vi "Dashboard custom_bartender&global&gripper&camera.vi"() -> ()   [LabVIEW 2017]
uses:
  C:/Users/IMR Lab/Documents/LabVIEW Data/UniversalRobotsSDK_LABView/LabVIEW/Examples/LabVIEW10/UnderAutomation.UniversalRobots.dll
  UnderAutomation.UniversalRobots.dll
  Global 1.vi
panel:
  out "RZ_havetogo":string
  out "RY_havetogo":string
  out "RX_havetogo":string
  out "Z_havetogo":string
  out "Y_havetogo":string
  out "X_havetogo":string
  out "data out":string
  out "TCPOffsetRZ":dbl
  out "TCPOffsetRY":dbl
  out "TCPOffsetRX":dbl
  out "TCPOffsetZ":dbl
  out "TCPOffsetY":dbl
  out "TCPOffsetX":dbl
  out "3rd Order":bool
  out "2nd Order":bool
  out "1st Order":bool
  in  "stop":bool
  in  "TCP switch (server)":bool
  out "Rx":dbl
  out "Rz":dbl
  out "Ry":dbl
  out "Enabled":bool
  out "Port":i32
  in  "Move to particular posture":bool
  in  "Move to Zero position":bool
  out "Connected":bool
  in  "Robot IP(192.168.112.182)":string
  out "Connect error":errorcluster
  in  "Power on\nRelease brake":bool
  in  "Power off":bool
  in  "Connect":bool
  in  "Send script":bool
  in  "Script to execute":string
  out "Powered on":bool
  out "X":dbl
  out "Y":dbl
  out "Z":dbl
  out "License state":string
  # "movel(p[-0.0753945, -0.304532, 0.314608, -0.194623, 2.71667, -1.00228], a= 0.5, v=0.25)"
  # "movej( get_inverse_kin(p[0.3138, 0.0814, 0.1647, 0.4226, -2.3876, -2.3851]),  a=0.5, v=0.25, t=0, r=0)"
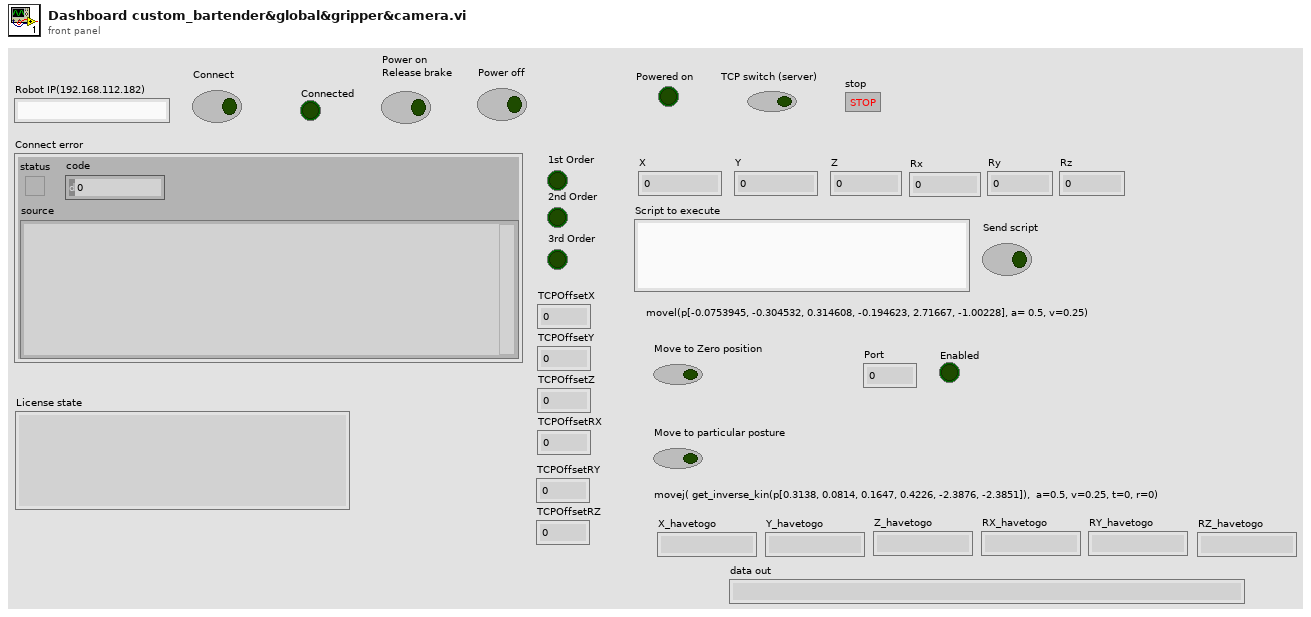
[diagram p1: front panel]
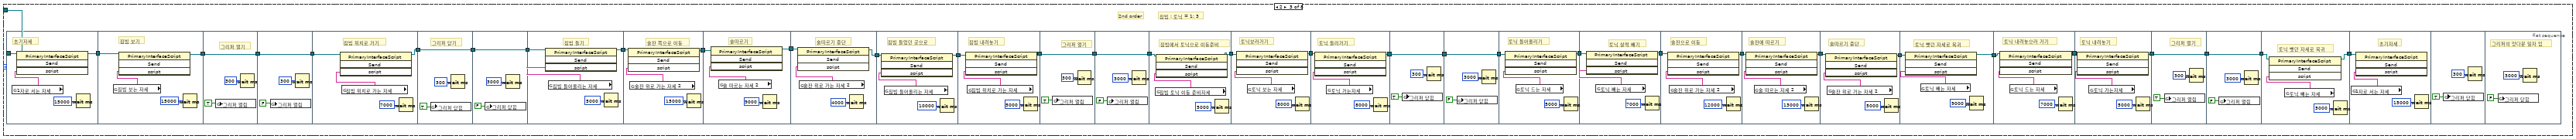
[diagram p5: hidden frame]
diagram:
  # "미니콜라 따르는 자세"
  # "술잔 중간지점 가는 자세"
  # "짐빔에서 토닉이동 준비 자세"
  # "술잔 따르는 자세2"
  # "술잔 위로 가는 자세2"
  # "토닉워터 뺴는 자세"
  # "토닉워 들어올리는 자세"
  # "토닉워터 가는 자세"
  # "토닉워터 보는 자세"
  # "짐빔 들어올리는 자세"
  # "짐빔로 가는 자세"
  # "짐빔 보는 자세"
  # "콜라 뺴는 자세"
  # "콜라 들어올리는 자세"
  # "콜라로 가는 자세"
  # "콜라 보는 자세"
  # "술잔 따르는 자세"
  # "술잔 위로 가는 자세"
  # "잭다니엘 들어올리는 자세"
  # "잭다니엘 위치로 가는 자세"
  # "잭다니엘 보는 자세"
  # "1자로 서는 자세"
  # "Example : Display power on status"
  # "Create a UR\ncobot instance"
  # "Show license state"
  # "Register your confidential license key to exit\ntrial period and use this library forever"
  # "Power off when button is clicked"
  # "Power on and release brake when button is clicked"
  # "Get your UR Dashboard interface"
  n1 = global write "Global 1.vi" "미니콜라 따르는 자세"("movej([-0.0902,-1.8120,-1.9241,-3.5769,6.2827,8.4658], a=0.5, v=0.25, t=0, r=0)") -> ()
  n2 = global write "Global 1.vi" "술잔 중간지점"("movej([-0.2173,-1.9485,-1.6874,-3.9352,6.2671,7.2276], a=0.5, v=0.25, t=0, r=0)") -> ()
  n3 = global write "Global 1.vi" "짐빔 토닉 이동 준비자세"("movej([-0.5421,-0.8131,0.8439,-0.0538,2.5052,5.9032], a=0.5, v=0.25, t=0, r=0)") -> ()
  n4 = global write "Global 1.vi" "잭다니엘 들어올리는 자세"("movej([0.8116,-2.0223,-1.2828,-3.0107,4.3284,5.9341], a=0.5, v=0.25, t=0, r=0)") -> ()
  n5 = global write "Global 1.vi" "잭다닐 위치로 가는 자세"("movej([0.8116,-2.3119,-1.606,-2.3958,4.3284,5.9341], a=0.5, v=0.25, t=0, r=0)") -> ()
  n6 = global write "Global 1.vi" "짐빔 들어올리는 자세"("movej([-0.5421,-0.8131,0.8439,-0.0538,2.5052,5.9032], a=0.5, v=0.25, t=0, r=0)") -> ()
  n7 = global write "Global 1.vi" "술잔 위로 가는 자세 2"("movej([0.0485,-1.6015,2.5780,-1.0382,-0.0520,5.3649], a=0.5, v=0.25, t=0, r=0)") -> ()
  n8 = global write "Global 1.vi" "1자로 서는 자세"("movej([3.1412,-1.5708,0,-1.5708,3.1412,5.8904], a=0.5, v=0.25, t=0, r=0)") -> ()
  n9 = global write "Global 1.vi" "짐빔 위치로 가는 자세"("movej([-0.5436,-0.4519,0.8428,-0.3534,2.6134,5.9032], a=0.5, v=0.25, t=0, r=0)") -> ()
  n10 = global write "Global 1.vi" "술잔 위로 가는 자세"("movej([-0.0903,-2.0548,-2.0169,-3.3289,6.2826,7.4091], a=0.5, v=0.25, t=0, r=0)") -> ()
  n11 = global write "Global 1.vi" "잭다니엘 보는 자세"("movej([0,-2.2170,-1.4226,-2.2842,3.1412,6.2832], a=0.5, v=0.25, t=0, r=0)") -> ()
  n12 = global write "Global 1.vi" "콜라 빼는 자세"("movej([0.8789,-1.5237,-2.1070,-2.6679, 3.9917,5.9085], a=0.5, v=0.25, t=0, r=0)") -> ()
  n13 = global write "Global 1.vi" "콜라 드는 자세"("movej([1.2020,-1.8452,-1.7403,-2.7082,4.3162,5.9158], a=0.5, v=0.25, t=0, r=0)") -> ()
  n14 = global write "Global 1.vi" "콜라 보는 자세"("movej([0,-1.8110,-2.1684,-2.3033,3.1543,5.9213], a=0.5, v=0.25, t=0, r=0)") -> ()
  n15 = global write "Global 1.vi" "콜라로 가는자세"("movej([1.2020,-2.166,-1.9385,-2.1863,4.3172,5.9210], a=0.5, v=0.25, t=0, r=0)") -> ()
  n16 = global write "Global 1.vi" "토닉 빼는 자세"("movej([-0.5277,-1.5104,1.5889,-0.0548,2.5728,5.9025], a=0.5, v=0.25, t=0, r=0)") -> ()
  n17 = global write "Global 1.vi" "술 따르는 자세 2"("movej([0.0412,-1.9708,2.4700,-1.0157,-0.0618,4.8998], a=0.5, v=0.25, t=0, r=0)") -> ()
  n18 = global write "Global 1.vi" "짐빔 보는 자세"("movej([-0.0364,-0.6154,0.9421,-0.3291,3.1047,5.9020], a=0.5, v=0.25, t=0, r=0)") -> ()
  n19 = global write "Global 1.vi" "토닉 드는 자세"("movej([-1.0311,-1.1460,1.5830,-0.4348,2.0708,5.9048], a=0.5, v=0.25, t=0, r=0)") -> ()
  n20 = global write "Global 1.vi" "토닉 보는 자세"("movej([-0.4690,-1.1292,2.1508,-1.0119,2.6124,5.9032], a=0.5, v=0.25, t=0, r=0)") -> ()
  n21 = global write "Global 1.vi" "술 따르는 자세"("movej([-0.0902,-1.9024,-1.9241,-3.5769,6.2827,8.4692], a=0.5, v=0.25, t=0, r=0)") -> ()
  n22 = global write "Global 1.vi" "토닉 가는자세"("movej([-0.9924,-0.8742,1.7459,-0.8837,2.0958,5.9048], a=0.5, v=0.25, t=0, r=0)") -> ()
  n23 = constructor class="UR"() -> (reference out=w25:refnum<k24>)  [unwired: 3 in, 2 out]
  n24 = while {
    tunnel: w25 -> [w31]
    stop <- FALSE stop-if-true
    # "Connect to the robot when button is pressed"
    # "Show if primary interface is connected"
    # "Get your UR primary interface"
    n25 = property class="UR"(reference=w31) -> ("PrimaryInterface"=w34:refnum<k24>)  [unwired: 1 in, 2 out]
    n26 = Wait (ms)(milliseconds to wait=u32 50) -> ()  [unwired: 1 out]
    n27 = property class="PrimaryInterfaceClientInternal"(reference=w34) -> ("Connected"=w33:bool)  [unwired: 1 in, 2 out]
    "Connected" <- w33
    n28 = case shown="True" "Connect" {
      tunnel: w31 -> [_ w403]
      frame False {
      }
      frame True {
        n29 = flat-sequence {
          tunnel: w403 -> [w405]
          frame #0 {
            n30 = invoke class="UR" method="Connect"(reference=w405, "ip"="Robot IP(192.168.112.182)") -> (error out=→"Connect error":errorcluster)  [unwired: 2 in, 3 out]
          }
        }
      }
    }
    n31 = case shown="True" w33 {
      tunnel: w34 -> [_ w40]
      frame False {
      }
      frame True {
        # "Send URScript when button pressed"
        # "Example : Display current cartesian pose"
        n32 = property class="PrimaryInterfaceClientInternal"(reference=w40) -> ("Script"=w48:refnum<k24>)  [unwired: 1 in, 2 out]
        n33 = global read "Global 1.vi" "2nd Order"() -> (w51:bool)
        "2nd Order" <- w51
        n34 = global read "Global 1.vi" "3rd Order"() -> (w50:bool)
        "3rd Order" <- w50
        n35 = global read "Global 1.vi" "1st Order"() -> (w52:bool)
        "1st Order" <- w52
        n36 = Build Array(w52, w51, w50) -> (w53:bool[])
        n37 = Boolean Array To Number(Boolean array=w53) -> (number=w49:u32)
        n38 = case shown="1" w49 {
          tunnel: w48 -> [_ w102 w238 _ _ _ _ _]
          frame 0, Default {
          }
          frame 1 {
            # "잭다 : 콜라 = 1 : 3"
            # "1st order"
            n39 = flat-sequence {
              tunnel: w102 -> [w106]
              tunnel: [w105] -> w101
              tunnel: w101 -> [w110]
              tunnel: [w108] -> w93
              tunnel: w93 -> [w113]
              tunnel: [w113] -> w91
              tunnel: w91 -> [w116]
              tunnel: [w116] -> w90
              tunnel: w90 -> [w120]
              tunnel: [w117] -> w92
              tunnel: w92 -> [w123]
              tunnel: [w123] -> w89
              tunnel: w89 -> [w126]
              tunnel: [w126] -> w88
              tunnel: w88 -> [w128]
              tunnel: [w127] -> w75
              tunnel: w75 -> [w132]
              tunnel: [w131] -> w74
              tunnel: w74 -> [w136]
              tunnel: [w135] -> w100
              tunnel: w100 -> [w141]
              tunnel: [w139] -> w99
              tunnel: w99 -> [w144]
              tunnel: [w143] -> w73
              tunnel: w73 -> [w148]
              tunnel: [w147] -> w72
              tunnel: [w151] -> w98
              tunnel: w72 -> [w153]
              tunnel: w98 -> [w156]
              tunnel: [w155] -> w87
              tunnel: w87 -> [w161]
              tunnel: [w161] -> w86
              tunnel: w86 -> [w164]
              tunnel: [w164] -> w85
              tunnel: w85 -> [w166]
              tunnel: [w165] -> w97
              tunnel: w97 -> [w170]
              tunnel: [w169] -> w84
              tunnel: w84 -> [w175]
              tunnel: [w175] -> w83
              tunnel: w83 -> [w178]
              tunnel: [w178] -> w82
              tunnel: w82 -> [w180]
              tunnel: [w179] -> w81
              tunnel: w81 -> [w184]
              tunnel: [w183] -> w71
              tunnel: w71 -> [w188]
              tunnel: [w187] -> w70
              tunnel: w70 -> [w192]
              tunnel: [w191] -> w96
              tunnel: w96 -> [w196]
              tunnel: [w195] -> w95
              tunnel: w95 -> [w200]
              tunnel: [w199] -> w69
              tunnel: w69 -> [w204]
              tunnel: [w203] -> w68
              tunnel: w68 -> [w208]
              tunnel: [w207] -> w80
              tunnel: w80 -> [w212]
              tunnel: [w211] -> w94
              tunnel: w94 -> [w216]
              tunnel: [w215] -> w78
              tunnel: [w219] -> w79
              tunnel: w78 -> [w219]
              tunnel: [w222] -> w77
              tunnel: w79 -> [w222]
              tunnel: w77 -> [w226]
              tunnel: [w225] -> w76
              tunnel: w76 -> [w229]
              frame #0 {
                # "초기자세"
                n40 = global read "Global 1.vi" "1자로 서는 자세"() -> (w104:string)
                n41 = invoke class="PrimaryInterfaceScript" method="Send"(reference=w106, "script"=w104) -> (reference out=w105:refnum<k24>)  [unwired: 2 in, 3 out]
                n42 = Wait (ms)(milliseconds to wait=u32 15000) -> ()  [unwired: 1 out]
              }
              frame #1 {
                # "잭다니엘 보기"
                n43 = global read "Global 1.vi" "잭다니엘 보는 자세"() -> (w109:string)
                n44 = invoke class="PrimaryInterfaceScript" method="Send"(reference=w110, "script"=w109) -> (reference out=w108:refnum<k24>)  [unwired: 2 in, 3 out]
                n45 = Wait (ms)(milliseconds to wait=u32 15000) -> ()  [unwired: 1 out]
              }
              frame #2 {
                # "그리퍼 열기"
                n46 = global write "Global 1.vi" "그리퍼 열림"(TRUE ("그리퍼 열림")) -> ()
                n47 = Wait (ms)(milliseconds to wait=u32 300) -> ()  [unwired: 1 out]
              }
              frame #3 {
                n48 = global write "Global 1.vi" "그리퍼 열림"(FALSE ("그리퍼 열림")) -> ()
                n49 = Wait (ms)(milliseconds to wait=u32 300) -> ()  [unwired: 1 out]
              }
              frame #4 {
                # "잭다니엘 위치로 가기"
                n50 = global read "Global 1.vi" "잭다닐 위치로 가는 자세"() -> (w119:string)
                n51 = invoke class="PrimaryInterfaceScript" method="Send"(reference=w120, "script"=w119) -> (reference out=w117:refnum<k24>)  [unwired: 2 in, 3 out]
                n52 = Wait (ms)(milliseconds to wait=u32 7000) -> ()  [unwired: 1 out]
              }
              frame #5 {
                # "그리퍼 닫기"
                n53 = global write "Global 1.vi" "그리퍼 닫힘"(TRUE ("그리퍼 열림")) -> ()
                n54 = Wait (ms)(milliseconds to wait=u32 300) -> ()  [unwired: 1 out]
              }
              frame #6 {
                n55 = global write "Global 1.vi" "그리퍼 닫힘"(FALSE ("그리퍼 열림")) -> ()
                n56 = Wait (ms)(milliseconds to wait=u32 3000) -> ()  [unwired: 1 out]
              }
              frame #7 {
                # "잭다니엘 들기"
                n57 = global read "Global 1.vi" "잭다니엘 들어올리는 자세"() -> (w130:string)
                n58 = invoke class="PrimaryInterfaceScript" method="Send"(reference=w128, "script"=w130) -> (reference out=w127:refnum<k24>)  [unwired: 2 in, 3 out]
                n59 = Wait (ms)(milliseconds to wait=u32 3000) -> ()  [unwired: 1 out]
              }
              frame #8 {
                # "술잔 중간지점으로 이동"
                n60 = global read "Global 1.vi" "술잔 중간지점"() -> (w133:string)
                n61 = invoke class="PrimaryInterfaceScript" method="Send"(reference=w132, "script"=w133) -> (reference out=w131:refnum<k24>)  [unwired: 2 in, 3 out]
                n62 = Wait (ms)(milliseconds to wait=u32 15000) -> ()  [unwired: 1 out]
              }
              frame #9 {
                # "술잔 쪽으로 이동"
                n63 = global read "Global 1.vi" "술잔 위로 가는 자세"() -> (w137:string)
                n64 = invoke class="PrimaryInterfaceScript" method="Send"(reference=w136, "script"=w137) -> (reference out=w135:refnum<k24>)  [unwired: 2 in, 3 out]
                n65 = Wait (ms)(milliseconds to wait=u32 5000) -> ()  [unwired: 1 out]
              }
              frame #10 {
                # "술따르기"
                n66 = global read "Global 1.vi" "술 따르는 자세"() -> (w140:string)
                n67 = invoke class="PrimaryInterfaceScript" method="Send"(reference=w141, "script"=w140) -> (reference out=w139:refnum<k24>)  [unwired: 2 in, 3 out]
                n68 = Wait (ms)(milliseconds to wait=u32 9000) -> ()  [unwired: 1 out]
              }
              frame #11 {
                # "술따르기 중단"
                n69 = global read "Global 1.vi" "술잔 위로 가는 자세"() -> (w145:string)
                n70 = invoke class="PrimaryInterfaceScript" method="Send"(reference=w144, "script"=w145) -> (reference out=w143:refnum<k24>)  [unwired: 2 in, 3 out]
                n71 = Wait (ms)(milliseconds to wait=u32 4000) -> ()  [unwired: 1 out]
              }
              frame #12 {
                # "술잔 중간지점으로 이동"
                n72 = global read "Global 1.vi" "술잔 중간지점"() -> (w149:string)
                n73 = invoke class="PrimaryInterfaceScript" method="Send"(reference=w148, "script"=w149) -> (reference out=w147:refnum<k24>)  [unwired: 2 in, 3 out]
                n74 = Wait (ms)(milliseconds to wait=u32 7000) -> ()  [unwired: 1 out]
              }
              frame #13 {
                # "잭다니엘 들었던 곳으로"
                n75 = global read "Global 1.vi" "잭다니엘 들어올리는 자세"() -> (w152:string)
                n76 = invoke class="PrimaryInterfaceScript" method="Send"(reference=w153, "script"=w152) -> (reference out=w151:refnum<k24>)  [unwired: 2 in, 3 out]
                n77 = Wait (ms)(milliseconds to wait=u32 10000) -> ()  [unwired: 1 out]
              }
              frame #14 {
                # "잭다니엘 내려놓기"
                n78 = global read "Global 1.vi" "잭다닐 위치로 가는 자세"() -> (w158:string)
                n79 = invoke class="PrimaryInterfaceScript" method="Send"(reference=w156, "script"=w158) -> (reference out=w155:refnum<k24>)  [unwired: 2 in, 3 out]
                n80 = Wait (ms)(milliseconds to wait=u32 5000) -> ()  [unwired: 1 out]
              }
              frame #15 {
                # "그리퍼 열기"
                n81 = global write "Global 1.vi" "그리퍼 열림"(TRUE ("그리퍼 열림")) -> ()
                n82 = Wait (ms)(milliseconds to wait=u32 300) -> ()  [unwired: 1 out]
              }
              frame #16 {
                n83 = global write "Global 1.vi" "그리퍼 열림"(FALSE ("그리퍼 열림")) -> ()
                n84 = Wait (ms)(milliseconds to wait=u32 3000) -> ()  [unwired: 1 out]
              }
              frame #17 {
                # "콜라보러가기"
                n85 = global read "Global 1.vi" "콜라 보는 자세"() -> (w168:string)
                n86 = invoke class="PrimaryInterfaceScript" method="Send"(reference=w166, "script"=w168) -> (reference out=w165:refnum<k24>)  [unwired: 2 in, 3 out]
                n87 = Wait (ms)(milliseconds to wait=u32 8000) -> ()  [unwired: 1 out]
              }
              frame #18 {
                # "콜라 들러가기"
                n88 = global read "Global 1.vi" "콜라로 가는자세"() -> (w172:string)
                n89 = invoke class="PrimaryInterfaceScript" method="Send"(reference=w170, "script"=w172) -> (reference out=w169:refnum<k24>)  [unwired: 2 in, 3 out]
                n90 = Wait (ms)(milliseconds to wait=u32 8000) -> ()  [unwired: 1 out]
              }
              frame #19 {
                n91 = global write "Global 1.vi" "그리퍼 닫힘"(TRUE ("그리퍼 열림")) -> ()
                n92 = Wait (ms)(milliseconds to wait=u32 300) -> ()  [unwired: 1 out]
              }
              frame #20 {
                n93 = global write "Global 1.vi" "그리퍼 닫힘"(FALSE ("그리퍼 열림")) -> ()
                n94 = Wait (ms)(milliseconds to wait=u32 3000) -> ()  [unwired: 1 out]
              }
              frame #21 {
                # "콜라 들어올리기"
                n95 = global read "Global 1.vi" "콜라 드는 자세"() -> (w182:string)
                n96 = invoke class="PrimaryInterfaceScript" method="Send"(reference=w180, "script"=w182) -> (reference out=w179:refnum<k24>)  [unwired: 2 in, 3 out]
                n97 = Wait (ms)(milliseconds to wait=u32 5000) -> ()  [unwired: 1 out]
              }
              frame #22 {
                # "콜라 살짝 빼기"
                n98 = global read "Global 1.vi" "콜라 빼는 자세"() -> (w186:string)
                n99 = invoke class="PrimaryInterfaceScript" method="Send"(reference=w184, "script"=w186) -> (reference out=w183:refnum<k24>)  [unwired: 2 in, 3 out]
                n100 = Wait (ms)(milliseconds to wait=u32 5000) -> ()  [unwired: 1 out]
              }
              frame #23 {
                # "술잔 중간지점으로 이동"
                n101 = global read "Global 1.vi" "술잔 중간지점"() -> (w189:string)
                n102 = invoke class="PrimaryInterfaceScript" method="Send"(reference=w188, "script"=w189) -> (reference out=w187:refnum<k24>)  [unwired: 2 in, 3 out]
                n103 = Wait (ms)(milliseconds to wait=u32 15000) -> ()  [unwired: 1 out]
              }
              frame #24 {
                # "술잔으로 이동"
                n104 = global read "Global 1.vi" "술잔 위로 가는 자세"() -> (w194:string)
                n105 = invoke class="PrimaryInterfaceScript" method="Send"(reference=w192, "script"=w194) -> (reference out=w191:refnum<k24>)  [unwired: 2 in, 3 out]
                n106 = Wait (ms)(milliseconds to wait=u32 5000) -> ()  [unwired: 1 out]
              }
              frame #25 {
                # "미니콜라에 따르기"
                n107 = global read "Global 1.vi" "미니콜라 따르는 자세"() -> (w198:string)
                n108 = invoke class="PrimaryInterfaceScript" method="Send"(reference=w196, "script"=w198) -> (reference out=w195:refnum<k24>)  [unwired: 2 in, 3 out]
                n109 = Wait (ms)(milliseconds to wait=u32 11000) -> ()  [unwired: 1 out]
              }
              frame #26 {
                # "술따르기 중단"
                n110 = global read "Global 1.vi" "술잔 위로 가는 자세"() -> (w202:string)
                n111 = invoke class="PrimaryInterfaceScript" method="Send"(reference=w200, "script"=w202) -> (reference out=w199:refnum<k24>)  [unwired: 2 in, 3 out]
                n112 = Wait (ms)(milliseconds to wait=u32 5000) -> ()  [unwired: 1 out]
              }
              frame #27 {
                # "술잔 중간지점으로 이동"
                n113 = global read "Global 1.vi" "술잔 중간지점"() -> (w205:string)
                n114 = invoke class="PrimaryInterfaceScript" method="Send"(reference=w204, "script"=w205) -> (reference out=w203:refnum<k24>)  [unwired: 2 in, 3 out]
                n115 = Wait (ms)(milliseconds to wait=u32 7000) -> ()  [unwired: 1 out]
              }
              frame #28 {
                # "콜라 뻇던 자세로 복귀"
                n116 = global read "Global 1.vi" "콜라 빼는 자세"() -> (w209:string)
                n117 = invoke class="PrimaryInterfaceScript" method="Send"(reference=w208, "script"=w209) -> (reference out=w207:refnum<k24>)  [unwired: 2 in, 3 out]
                n118 = Wait (ms)(milliseconds to wait=u32 7000) -> ()  [unwired: 1 out]
              }
              frame #29 {
                # "콜라 내려놓으러 가기"
                n119 = global read "Global 1.vi" "콜라 드는 자세"() -> (w214:string)
                n120 = invoke class="PrimaryInterfaceScript" method="Send"(reference=w212, "script"=w214) -> (reference out=w211:refnum<k24>)  [unwired: 2 in, 3 out]
                n121 = Wait (ms)(milliseconds to wait=u32 10000) -> ()  [unwired: 1 out]
              }
              frame #30 {
                # "콜라 내려놓기"
                n122 = global read "Global 1.vi" "콜라로 가는자세"() -> (w218:string)
                n123 = invoke class="PrimaryInterfaceScript" method="Send"(reference=w216, "script"=w218) -> (reference out=w215:refnum<k24>)  [unwired: 2 in, 3 out]
                n124 = Wait (ms)(milliseconds to wait=u32 5000) -> ()  [unwired: 1 out]
              }
              frame #31 {
                # "그리퍼 열기"
                n125 = global write "Global 1.vi" "그리퍼 열림"(TRUE ("그리퍼 열림")) -> ()
                n126 = Wait (ms)(milliseconds to wait=u32 300) -> ()  [unwired: 1 out]
              }
              frame #32 {
                n127 = global write "Global 1.vi" "그리퍼 열림"(FALSE ("그리퍼 열림")) -> ()
                n128 = Wait (ms)(milliseconds to wait=u32 3000) -> ()  [unwired: 1 out]
              }
              frame #33 {
                # "콜라 뻇던 자세로 복귀"
                n129 = global read "Global 1.vi" "콜라 빼는 자세"() -> (w227:string)
                n130 = invoke class="PrimaryInterfaceScript" method="Send"(reference=w226, "script"=w227) -> (reference out=w225:refnum<k24>)  [unwired: 2 in, 3 out]
                n131 = Wait (ms)(milliseconds to wait=u32 5000) -> ()  [unwired: 1 out]
              }
              frame #34 {
                # "초기자세"
                n132 = global read "Global 1.vi" "1자로 서는 자세"() -> (w231:string)
                n133 = invoke class="PrimaryInterfaceScript" method="Send"(reference=w229, "script"=w231) -> ()  [unwired: 2 in, 4 out]
                n134 = Wait (ms)(milliseconds to wait=u32 15000) -> ()  [unwired: 1 out]
              }
              frame #35 {
                n135 = global write "Global 1.vi" "그리퍼 닫힘"(TRUE ("그리퍼 열림")) -> ()
                n136 = Wait (ms)(milliseconds to wait=u32 300) -> ()  [unwired: 1 out]
              }
              frame #36 {
                # "그리퍼의 앙다문 일자 입"
                n137 = global write "Global 1.vi" "그리퍼 닫힘"(FALSE ("그리퍼 열림")) -> ()
                n138 = Wait (ms)(milliseconds to wait=u32 3000) -> ()  [unwired: 1 out]
              }
            }
          }
          frame 2 {
            # "짐빔 : 토닉 = 1: 3"
            # "2nd order"
            n139 = flat-sequence {
              tunnel: w238 -> [w271]
              tunnel: [w270] -> w267
              tunnel: w267 -> [w275]
              tunnel: [w273] -> w266
              tunnel: w266 -> [w278]
              tunnel: [w278] -> w265
              tunnel: w265 -> [w281]
              tunnel: [w281] -> w264
              tunnel: w264 -> [w285]
              tunnel: [w282] -> w263
              tunnel: w263 -> [w288]
              tunnel: [w288] -> w262
              tunnel: w262 -> [w291]
              tunnel: [w291] -> w261
              tunnel: w261 -> [w293]
              tunnel: [w292] -> w260
              tunnel: w260 -> [w297]
              tunnel: [w296] -> w259
              tunnel: w259 -> [w302]
              tunnel: [w300] -> w258
              tunnel: w258 -> [w305]
              tunnel: [w304] -> w257
              tunnel: w257 -> [w310]
              tunnel: [w308] -> w256
              tunnel: w256 -> [w313]
              tunnel: [w312] -> w255
              tunnel: w255 -> [w318]
              tunnel: [w318] -> w254
              tunnel: w254 -> [w321]
              tunnel: [w321] -> w237
              tunnel: w237 -> [w323]
              tunnel: [w322] -> w236
              tunnel: [w326] -> w253
              tunnel: w236 -> [w327]
              tunnel: w253 -> [w331]
              tunnel: [w330] -> w252
              tunnel: w252 -> [w336]
              tunnel: [w336] -> w251
              tunnel: w251 -> [w339]
              tunnel: [w339] -> w250
              tunnel: w250 -> [w341]
              tunnel: [w340] -> w249
              tunnel: w249 -> [w345]
              tunnel: [w344] -> w248
              tunnel: w248 -> [w349]
              tunnel: [w348] -> w247
              tunnel: w247 -> [w353]
              tunnel: [w352] -> w246
              tunnel: w246 -> [w357]
              tunnel: [w356] -> w245
              tunnel: w245 -> [w361]
              tunnel: [w360] -> w244
              tunnel: w244 -> [w365]
              tunnel: [w364] -> w243
              tunnel: w243 -> [w369]
              tunnel: [w368] -> w242
              tunnel: [w372] -> w241
              tunnel: w242 -> [w372]
              tunnel: [w375] -> w240
              tunnel: w241 -> [w375]
              tunnel: w240 -> [w379]
              tunnel: [w378] -> w239
              tunnel: w239 -> [w382]
              frame #0 {
                # "초기자세"
                n140 = global read "Global 1.vi" "1자로 서는 자세"() -> (w269:string)
                n141 = invoke class="PrimaryInterfaceScript" method="Send"(reference=w271, "script"=w269) -> (reference out=w270:refnum<k24>)  [unwired: 2 in, 3 out]
                n142 = Wait (ms)(milliseconds to wait=u32 15000) -> ()  [unwired: 1 out]
              }
              frame #1 {
                # "짐빔 보기"
                n143 = global read "Global 1.vi" "짐빔 보는 자세"() -> (w274:string)
                n144 = invoke class="PrimaryInterfaceScript" method="Send"(reference=w275, "script"=w274) -> (reference out=w273:refnum<k24>)  [unwired: 2 in, 3 out]
                n145 = Wait (ms)(milliseconds to wait=u32 15000) -> ()  [unwired: 1 out]
              }
              frame #2 {
                # "그리퍼 열기"
                n146 = global write "Global 1.vi" "그리퍼 열림"(TRUE ("그리퍼 열림")) -> ()
                n147 = Wait (ms)(milliseconds to wait=u32 300) -> ()  [unwired: 1 out]
              }
              frame #3 {
                n148 = global write "Global 1.vi" "그리퍼 열림"(FALSE ("그리퍼 열림")) -> ()
                n149 = Wait (ms)(milliseconds to wait=u32 300) -> ()  [unwired: 1 out]
              }
              frame #4 {
                # "짐빔 위치로 가기"
                n150 = global read "Global 1.vi" "짐빔 위치로 가는 자세"() -> (w284:string)
                n151 = invoke class="PrimaryInterfaceScript" method="Send"(reference=w285, "script"=w284) -> (reference out=w282:refnum<k24>)  [unwired: 2 in, 3 out]
                n152 = Wait (ms)(milliseconds to wait=u32 7000) -> ()  [unwired: 1 out]
              }
              frame #5 {
                # "그리퍼 닫기"
                n153 = global write "Global 1.vi" "그리퍼 닫힘"(TRUE ("그리퍼 열림")) -> ()
                n154 = Wait (ms)(milliseconds to wait=u32 300) -> ()  [unwired: 1 out]
              }
              frame #6 {
                n155 = global write "Global 1.vi" "그리퍼 닫힘"(FALSE ("그리퍼 열림")) -> ()
                n156 = Wait (ms)(milliseconds to wait=u32 3000) -> ()  [unwired: 1 out]
              }
              frame #7 {
                # "짐빔 들기"
                n157 = global read "Global 1.vi" "짐빔 들어올리는 자세"() -> (w295:string)
                n158 = invoke class="PrimaryInterfaceScript" method="Send"(reference=w293, "script"=w295) -> (reference out=w292:refnum<k24>)  [unwired: 2 in, 3 out]
                n159 = Wait (ms)(milliseconds to wait=u32 5000) -> ()  [unwired: 1 out]
              }
              frame #8 {
                # "술잔 쪽으로 이동"
                n160 = global read "Global 1.vi" "술잔 위로 가는 자세 2"() -> (w298:string)
                n161 = invoke class="PrimaryInterfaceScript" method="Send"(reference=w297, "script"=w298) -> (reference out=w296:refnum<k24>)  [unwired: 2 in, 3 out]
                n162 = Wait (ms)(milliseconds to wait=u32 15000) -> ()  [unwired: 1 out]
              }
              frame #9 {
                # "술따르기"
                n163 = global read "Global 1.vi" "술 따르는 자세 2"() -> (w301:string)
                n164 = invoke class="PrimaryInterfaceScript" method="Send"(reference=w302, "script"=w301) -> (reference out=w300:refnum<k24>)  [unwired: 2 in, 3 out]
                n165 = Wait (ms)(milliseconds to wait=u32 9000) -> ()  [unwired: 1 out]
              }
              frame #10 {
                # "술따르기 중단"
                n166 = global read "Global 1.vi" "술잔 위로 가는 자세 2"() -> (w306:string)
                n167 = invoke class="PrimaryInterfaceScript" method="Send"(reference=w305, "script"=w306) -> (reference out=w304:refnum<k24>)  [unwired: 2 in, 3 out]
                n168 = Wait (ms)(milliseconds to wait=u32 4000) -> ()  [unwired: 1 out]
              }
              frame #11 {
                # "짐빔 들었던 곳으로"
                n169 = global read "Global 1.vi" "짐빔 들어올리는 자세"() -> (w309:string)
                n170 = invoke class="PrimaryInterfaceScript" method="Send"(reference=w310, "script"=w309) -> (reference out=w308:refnum<k24>)  [unwired: 2 in, 3 out]
                n171 = Wait (ms)(milliseconds to wait=u32 10000) -> ()  [unwired: 1 out]
              }
              frame #12 {
                # "짐빔 내려놓기"
                n172 = global read "Global 1.vi" "짐빔 위치로 가는 자세"() -> (w315:string)
                n173 = invoke class="PrimaryInterfaceScript" method="Send"(reference=w313, "script"=w315) -> (reference out=w312:refnum<k24>)  [unwired: 2 in, 3 out]
                n174 = Wait (ms)(milliseconds to wait=u32 5000) -> ()  [unwired: 1 out]
              }
              frame #13 {
                # "그리퍼 열기"
                n175 = global write "Global 1.vi" "그리퍼 열림"(TRUE ("그리퍼 열림")) -> ()
                n176 = Wait (ms)(milliseconds to wait=u32 300) -> ()  [unwired: 1 out]
              }
              frame #14 {
                n177 = global write "Global 1.vi" "그리퍼 열림"(FALSE ("그리퍼 열림")) -> ()
                n178 = Wait (ms)(milliseconds to wait=u32 3000) -> ()  [unwired: 1 out]
              }
              frame #15 {
                # "짐빔에서 토닉으로 이동준비"
                n179 = global read "Global 1.vi" "짐빔 토닉 이동 준비자세"() -> (w325:string)
                n180 = invoke class="PrimaryInterfaceScript" method="Send"(reference=w323, "script"=w325) -> (reference out=w322:refnum<k24>)  [unwired: 2 in, 3 out]
                n181 = Wait (ms)(milliseconds to wait=u32 5000) -> ()  [unwired: 1 out]
              }
              frame #16 {
                # "토닉보러가기"
                n182 = global read "Global 1.vi" "토닉 보는 자세"() -> (w329:string)
                n183 = invoke class="PrimaryInterfaceScript" method="Send"(reference=w327, "script"=w329) -> (reference out=w326:refnum<k24>)  [unwired: 2 in, 3 out]
                n184 = Wait (ms)(milliseconds to wait=u32 8000) -> ()  [unwired: 1 out]
              }
              frame #17 {
                # "토닉 들러가기"
                n185 = global read "Global 1.vi" "토닉 가는자세"() -> (w333:string)
                n186 = invoke class="PrimaryInterfaceScript" method="Send"(reference=w331, "script"=w333) -> (reference out=w330:refnum<k24>)  [unwired: 2 in, 3 out]
                n187 = Wait (ms)(milliseconds to wait=u32 8000) -> ()  [unwired: 1 out]
              }
              frame #18 {
                n188 = global write "Global 1.vi" "그리퍼 닫힘"(TRUE ("그리퍼 열림")) -> ()
                n189 = Wait (ms)(milliseconds to wait=u32 300) -> ()  [unwired: 1 out]
              }
              frame #19 {
                n190 = global write "Global 1.vi" "그리퍼 닫힘"(FALSE ("그리퍼 열림")) -> ()
                n191 = Wait (ms)(milliseconds to wait=u32 3000) -> ()  [unwired: 1 out]
              }
              frame #20 {
                # "토닉 들어올리기"
                n192 = global read "Global 1.vi" "토닉 드는 자세"() -> (w343:string)
                n193 = invoke class="PrimaryInterfaceScript" method="Send"(reference=w341, "script"=w343) -> (reference out=w340:refnum<k24>)  [unwired: 2 in, 3 out]
                n194 = Wait (ms)(milliseconds to wait=u32 5000) -> ()  [unwired: 1 out]
              }
              frame #21 {
                # "토닉 살짝 빼기"
                n195 = global read "Global 1.vi" "토닉 빼는 자세"() -> (w347:string)
                n196 = invoke class="PrimaryInterfaceScript" method="Send"(reference=w345, "script"=w347) -> (reference out=w344:refnum<k24>)  [unwired: 2 in, 3 out]
                n197 = Wait (ms)(milliseconds to wait=u32 7000) -> ()  [unwired: 1 out]
              }
              frame #22 {
                # "술잔으로 이동"
                n198 = global read "Global 1.vi" "술잔 위로 가는 자세 2"() -> (w351:string)
                n199 = invoke class="PrimaryInterfaceScript" method="Send"(reference=w349, "script"=w351) -> (reference out=w348:refnum<k24>)  [unwired: 2 in, 3 out]
                n200 = Wait (ms)(milliseconds to wait=u32 12000) -> ()  [unwired: 1 out]
              }
              frame #23 {
                # "술잔에 따르기"
                n201 = global read "Global 1.vi" "술 따르는 자세 2"() -> (w355:string)
                n202 = invoke class="PrimaryInterfaceScript" method="Send"(reference=w353, "script"=w355) -> (reference out=w352:refnum<k24>)  [unwired: 2 in, 3 out]
                n203 = Wait (ms)(milliseconds to wait=u32 13000) -> ()  [unwired: 1 out]
              }
              frame #24 {
                # "술따르기 중단"
                n204 = global read "Global 1.vi" "술잔 위로 가는 자세 2"() -> (w359:string)
                n205 = invoke class="PrimaryInterfaceScript" method="Send"(reference=w357, "script"=w359) -> (reference out=w356:refnum<k24>)  [unwired: 2 in, 3 out]
                n206 = Wait (ms)(milliseconds to wait=u32 5000) -> ()  [unwired: 1 out]
              }
              frame #25 {
                # "토닉 뻇던 자세로 복귀"
                n207 = global read "Global 1.vi" "토닉 빼는 자세"() -> (w362:string)
                n208 = invoke class="PrimaryInterfaceScript" method="Send"(reference=w361, "script"=w362) -> (reference out=w360:refnum<k24>)  [unwired: 2 in, 3 out]
                n209 = Wait (ms)(milliseconds to wait=u32 9000) -> ()  [unwired: 1 out]
              }
              frame #26 {
                # "토닉 내려놓으러 가기"
                n210 = global read "Global 1.vi" "토닉 드는 자세"() -> (w367:string)
                n211 = invoke class="PrimaryInterfaceScript" method="Send"(reference=w365, "script"=w367) -> (reference out=w364:refnum<k24>)  [unwired: 2 in, 3 out]
                n212 = Wait (ms)(milliseconds to wait=u32 7000) -> ()  [unwired: 1 out]
              }
              frame #27 {
                # "토닉 내려놓기"
                n213 = global read "Global 1.vi" "토닉 가는자세"() -> (w371:string)
                n214 = invoke class="PrimaryInterfaceScript" method="Send"(reference=w369, "script"=w371) -> (reference out=w368:refnum<k24>)  [unwired: 2 in, 3 out]
                n215 = Wait (ms)(milliseconds to wait=u32 5000) -> ()  [unwired: 1 out]
              }
              frame #28 {
                # "그리퍼 열기"
                n216 = global write "Global 1.vi" "그리퍼 열림"(TRUE ("그리퍼 열림")) -> ()
                n217 = Wait (ms)(milliseconds to wait=u32 300) -> ()  [unwired: 1 out]
              }
              frame #29 {
                n218 = global write "Global 1.vi" "그리퍼 열림"(FALSE ("그리퍼 열림")) -> ()
                n219 = Wait (ms)(milliseconds to wait=u32 3000) -> ()  [unwired: 1 out]
              }
              frame #30 {
                # "토닉 뻇던 자세로 복귀"
                n220 = global read "Global 1.vi" "토닉 빼는 자세"() -> (w380:string)
                n221 = invoke class="PrimaryInterfaceScript" method="Send"(reference=w379, "script"=w380) -> (reference out=w378:refnum<k24>)  [unwired: 2 in, 3 out]
                n222 = Wait (ms)(milliseconds to wait=u32 5000) -> ()  [unwired: 1 out]
              }
              frame #31 {
                # "초기자세"
                n223 = global read "Global 1.vi" "1자로 서는 자세"() -> (w384:string)
                n224 = invoke class="PrimaryInterfaceScript" method="Send"(reference=w382, "script"=w384) -> ()  [unwired: 2 in, 4 out]
                n225 = Wait (ms)(milliseconds to wait=u32 15000) -> ()  [unwired: 1 out]
              }
              frame #32 {
                n226 = global write "Global 1.vi" "그리퍼 닫힘"(TRUE ("그리퍼 열림")) -> ()
                n227 = Wait (ms)(milliseconds to wait=u32 300) -> ()  [unwired: 1 out]
              }
              frame #33 {
                # "그리퍼의 앙다문 일자 입"
                n228 = global write "Global 1.vi" "그리퍼 닫힘"(FALSE ("그리퍼 열림")) -> ()
                n229 = Wait (ms)(milliseconds to wait=u32 3000) -> ()  [unwired: 1 out]
              }
            }
          }
          frame 3 {
            # "multi order"
          }
          frame 4 {
            # "짐빔 : 우유 = 1 : 3"
            # "3rd order"
          }
          frame 5 {
            # "multi order"
          }
          frame 6 {
            # "multi order"
          }
          frame 7 {
            # "multi order"
          }
        }
        n230 = case shown="True" "Send script" {
          tunnel: w48 -> [_ w395]
          frame False {
          }
          frame True {
            n231 = flat-sequence {
              tunnel: w395 -> [w397]
              frame #0 {
                n232 = invoke class="PrimaryInterfaceScript" method="Send"(reference=w397, "script"="Script to execute") -> ()  [unwired: 2 in, 4 out]
              }
            }
          }
        }
        n233 = case shown="True" "Move to Zero position" {
          tunnel: w48 -> [_ w392]
          frame False {
          }
          frame True {
            n234 = flat-sequence {
              tunnel: w392 -> [w394]
              frame #0 {
                n235 = invoke class="PrimaryInterfaceScript" method="Send"(reference=w394, "script"="movej([3.1412,-1.5708,0,-1.5708,3.1412,5.8904], a=0.5, v=0.25, t=0, r=0)") -> ()  [unwired: 2 in, 4 out]
              }
            }
          }
        }
        n236 = case shown="True" "Move to particular posture" {
          tunnel: w48 -> [_ w389]
          frame False {
          }
          frame True {
            n237 = flat-sequence {
              tunnel: w389 -> [w391]
              frame #0 {
                n238 = invoke class="PrimaryInterfaceScript" method="Send"(reference=w391, "script"="movej([-1.5,-1.5,-2,-0.5,1.8,0], a=1.4, v=1.05, t=0, r=0)") -> ()  [unwired: 2 in, 4 out]
              }
            }
          }
        }
        n239 = property class="PrimaryInterfaceClientInternal"(reference=w40) -> ("RobotModeData"=w66:refnum<k24>)  [unwired: 1 in, 2 out]
        n240 = property class="PrimaryInterfaceClientInternal"(reference=w40) -> ("CartesianInfo"=w47:refnum<k24>)  [unwired: 1 in, 2 out]
        n241 = property class="RobotModeDataPackageEventArgs"(reference=w66) -> ("RobotPowerOn"=→"Powered on":bool)  [unwired: 1 in, 2 out]
        n242 = constructor class="SocketCommunicationServer"() -> (reference out=w59:refnum<k24>)  [unwired: 3 in, 2 out]
        n243 = property class="SocketCommunicationServer"(reference=w59) -> ("Enabled"=→"Enabled":bool)  [unwired: 1 in, 2 out]
        n244 = property class="SocketCommunicationServer"(reference=w59) -> ("Port"=→"Port":i32)  [unwired: 1 in, 2 out]
        n245 = property class="CartesianInfoPackageEventArgs"(reference=w47) -> ("TCPOffsetX"=→"TCPOffsetX":dbl)  [unwired: 1 in, 2 out]
        n246 = property class="CartesianInfoPackageEventArgs"(reference=w47) -> ("TCPOffsetY"=→"TCPOffsetY":dbl)  [unwired: 1 in, 2 out]
        n247 = property class="CartesianInfoPackageEventArgs"(reference=w47) -> ("TCPOffsetRX"=→"TCPOffsetRX":dbl)  [unwired: 1 in, 2 out]
        n248 = property class="CartesianInfoPackageEventArgs"(reference=w47) -> ("TCPOffsetRY"=→"TCPOffsetRY":dbl)  [unwired: 1 in, 2 out]
        n249 = property class="CartesianInfoPackageEventArgs"(reference=w47) -> ("Y"=→"Y":dbl)  [unwired: 1 in, 2 out]
        n250 = property class="CartesianInfoPackageEventArgs"(reference=w47) -> ("TCPOffsetZ"=→"TCPOffsetZ":dbl)  [unwired: 1 in, 2 out]
        n251 = property class="CartesianInfoPackageEventArgs"(reference=w47) -> ("TCPOffsetRZ"=→"TCPOffsetRZ":dbl)  [unwired: 1 in, 2 out]
        n252 = property class="CartesianInfoPackageEventArgs"(reference=w47) -> ("Ry"=→"Ry":dbl)  [unwired: 1 in, 2 out]
        n253 = property class="CartesianInfoPackageEventArgs"(reference=w47) -> ("Z"=→"Z":dbl)  [unwired: 1 in, 2 out]
        n254 = property class="CartesianInfoPackageEventArgs"(reference=w47) -> ("Rz"=→"Rz":dbl)  [unwired: 1 in, 2 out]
        n255 = property class="CartesianInfoPackageEventArgs"(reference=w47) -> ("X"=→"X":dbl)  [unwired: 1 in, 2 out]
        n256 = property class="CartesianInfoPackageEventArgs"(reference=w47) -> ("Rx"=→"Rx":dbl)  [unwired: 1 in, 2 out]
      }
    }
    n257 = property class="UR"(reference=w31) -> ("Dashboard"=w35:refnum<k24>)  [unwired: 1 in, 2 out]
    n258 = case shown="True" "Power off" {
      tunnel: w35 -> [_ w398]
      frame False {
      }
      frame True {
        n259 = flat-sequence {
          tunnel: w398 -> [w399]
          frame #0 {
            n260 = invoke class="DashboardClientInternal" method="PowerOff"(reference=w399) -> ()  [unwired: 2 in, 3 out]
          }
        }
      }
    }
    n261 = case shown="True" "Power on\nRelease brake" {
      tunnel: w35 -> [_ w400]
      frame False {
      }
      frame True {
        n262 = flat-sequence {
          tunnel: w400 -> [w402]
          frame #0 {
            n263 = invoke class="DashboardClientInternal" method="PowerOn"(reference=w402) -> (reference out=w401:refnum<k24>)  [unwired: 2 in, 2 out]
            n264 = invoke class="DashboardClientInternal" method="ReleaseBrake"(reference=w401) -> ()  [unwired: 2 in, 3 out]
          }
        }
      }
    }
  }
  n265 = invoke class="UR" method="RegisterLicense"(reference=w25, "licensee"="your company name", "key"="") -> (reference out=w27:refnum<k24>)  [unwired: 2 in, 4 out]
  n266 = control-ref of="Script to execute"() -> (w24:refnum<vi>)
  n267 = property class="Str"(reference=w24, "Value"="movej([-1.5,-1.5,-2,-0.5,1.8,0], a=1.4, v=1.05, t=0, r=0)") -> ()  [unwired: 1 in, 2 out]
  n268 = property class="UR"(reference=w27) -> ("LicenseInfo"=w26:refnum<k24>)  [unwired: 1 in, 2 out]
  n269 = invoke class="LicenseInfo" method="ToString"(reference=w26) -> ("ToString"=→"License state":string)  [unwired: 2 in, 2 out]
  n270 = while {
    stop <- "stop" stop-if-true
    n271 = case shown="True" "TCP switch (server)" {
      frame False {
      }
      frame True {
        w414 = 4 ("length (rest)")
        n272 = TCP Open Connection(address="localhost", remote port or service name=u16 9999) -> (connection ID=w426:refnum<k5>, error out=w425:errorcluster)  [unwired: 3 in]
        n273 = TCP Read(connection ID=w426, error in (no error)=w425) -> (connection ID out=w424:refnum<k5>, data out=w415:string, error out=w423:errorcluster)  [unwired: 3 in]
        "data out" <- w415
        n274 = String Subset(string=w415, offset (0)=8, length (rest)=w414) -> (substring=→"Z_havetogo":string)
        n275 = String Subset(string=w415, offset (0)=12, length (rest)=w414) -> (substring=→"RX_havetogo":string)
        n276 = String Subset(string=w415, offset (0)=4, length (rest)=w414) -> (substring=→"Y_havetogo":string)
        n277 = String Subset(string=w415, offset (0)=0, length (rest)=w414) -> (substring=→"X_havetogo":string)
        n278 = String Subset(string=w415, offset (0)=20, length (rest)=w414) -> (substring=→"RZ_havetogo":string)
        n279 = String Subset(string=w415, offset (0)=16, length (rest)=w414) -> (substring=→"RY_havetogo":string)
        n280 = TCP Close Connection(connection ID=w424, error in (no error)=w423) -> ()  [unwired: 1 in, 2 out]
      }
    }
  }
